vi "DeQueue Trigger.vi"(0 "Queue in":refnum<queue>, 9 "Timeout (0)":i32, 11 "error in (no error)":errorcluster) -> (4 "Queue out":refnum<queue>, 6 "System Triggers":T1, 10 "Trigger Data":variant, 15 "error out":errorcluster)   [LabVIEW 2014, in "TLB` Template.lvlib"]
uses:
  TLB` Template.lvlib
  System Trigger.ctl
  System Trigger Element.ctl
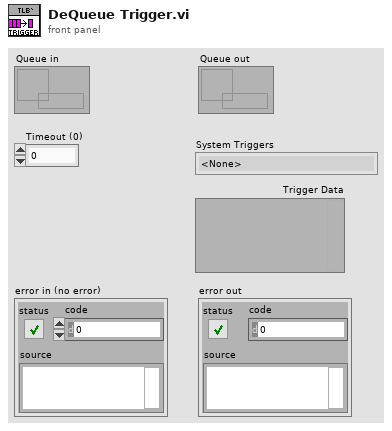
[diagram p1: front panel]
types:
  T1 = typedef "TLB` Template.lvlib/System Trigger.ctl" = enum16{"<None>", "Cache User Parameters", "Close Application"}
  T2 = typedef "TLB` Template.lvlib/System Trigger Element.ctl" = cluster{"System Triggers":T1, "Trigger Data":variant}
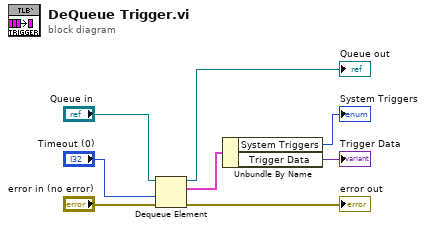
[diagram p0: block diagram]
diagram:
  n1 = Dequeue Element(queue="Queue in", timeout in ms (-1)="Timeout (0)", error in (no error)="error in (no error)") -> (queue out=→"Queue out":refnum<queue>, element=w3:T2, error out=→"error out":errorcluster)  [unwired: 1 out]
  n2 = Unbundle By Name(w3) -> ("System Triggers"=→"System Triggers":T1, "Trigger Data"=→"Trigger Data":variant)
